vi "FPGA Target 2.vi"() -> ()   [LabVIEW 2019]
uses:
  <vilib>/Platform/TimedLoop/XDataNode/wakeup.ctl
  <vilib>/Platform/TimedLoop/XDataNode/XDNodeRunTimeDep.lvlib
  <vilib>/Platform/TimedLoop/XDataNode/nitl_modes.ctl
  <vilib>/Platform/TimedLoop/XDataNode/timing_clust.ctl
  <vilib>/Platform/TimedLoop/XDataNode/XDataNode.xnode
  SubModules/Engine Simulation Toolkit FPGA IP/IP Source/APU/APU.lvlib
  <vilib>/rvi/DataTransferAndStorage/Container/XNode/niFpgaContainer.xnode
  Templates/FPGA Wizard Templates.lvlib
  SubModules/Engine Simulation Toolkit FPGA IP/IP Source/Digital Pattern Generation/Digital Pattern Generation.lvlib
  SubModules/Engine Simulation Toolkit FPGA IP/IP Source/Directional Speed/Directional Speed.lvlib
  SubModules/FPGA Addon Speciality IO/Source/Speciality FPGA IO.lvlib
  SubModules/Engine Simulation Toolkit FPGA IP/IP Source/ECU Event/Timing/ECU Event Timing.lvlib
  SubModules/Engine Simulation Toolkit FPGA IP/IP Source/ECU Event/Timing/Measure Events (Non-40MHz).vi
  SubModules/Engine Simulation Toolkit FPGA IP/IP Source/ECU Event/Timing/Capture Settings.ctl
  <vilib>/rvi/interface/RandomDataEmulation/nirviRandomDataFpgaReadWriteTemplate.vi
  SubModules/Engine Simulation Toolkit FPGA IP/IP Source/APU/Shared Settings.ctl
  SubModules/Engine Simulation Toolkit FPGA IP/IP Source/Version Token.ctl
  SubModules/Engine Simulation Toolkit FPGA IP/IP Source/Engine Simulation Toolkit.lvlib
  SubModules/Engine Simulation Toolkit FPGA IP/IP Source/APU/Settings.ctl
  SubModules/Engine Simulation Toolkit FPGA IP/IP Source/APU/Input.ctl
  SubModules/Engine Simulation Toolkit FPGA IP/IP Source/APU/Output.ctl
  SubModules/Engine Simulation Toolkit FPGA IP/IP Source/Digital Pattern Generation/Load Input.ctl
  SubModules/Engine Simulation Toolkit FPGA IP/IP Source/Directional Speed/Load Input.ctl
  SubModules/FPGA Addon Speciality IO/Source/Types/PWM.Generate.Digital.Settings.ctl
  SubModules/FPGA Addon Speciality IO/Source/Types/PWM.Measure.Digital.Settings.ctl
  SubModules/FPGA Addon Speciality IO/Source/Types/PWM.Measure.Digital.Measurement.ctl
  SubModules/FPGA Addon Speciality IO/Source/Types/Static.Measure.Digital.Settings.ctl
  SubModules/FPGA Addon Speciality IO/Source/Types/Static.Measure.Digital.Measurement.ctl
  SubModules/FPGA Addon Speciality IO/Source/Types/Static.Generate.Digital.Settings.ctl
  SubModules/Engine Simulation Toolkit FPGA IP/IP Source/Digital Pattern Generation/Settings.ctl
  SubModules/Engine Simulation Toolkit FPGA IP/IP Source/Digital Pattern Generation/Input.ctl
  SubModules/FPGA Addon Speciality IO/Source/Types/WSS.Generate.Digital.Settings.ctl
  SubModules/Engine Simulation Toolkit FPGA IP/IP Source/Directional Speed/Settings.ctl
  SubModules/Engine Simulation Toolkit FPGA IP/IP Source/Directional Speed/Input.ctl
  SubModules/Engine Simulation Toolkit FPGA IP/IP Source/ECU Event/Timing/Measure Settings.ctl
  SubModules/Engine Simulation Toolkit FPGA IP/IP Source/ECU Event/Timing/Measure Output.ctl
  SubModules/Engine Simulation Toolkit FPGA IP/IP Source/ECU Event/Timing/Capture Output.ctl
panel:
  out "capture.Cyl Inj 2.Event 4":T1
  out "capture.Cyl Inj 2.Event 3":T1
  out "capture.Cyl Inj 2.Event 2":T1
  out "capture.Cyl Inj 2.Event 1":T1
  out "status.Cyl Inj 2":T2
  in  "settings.Cyl Inj 2":T3
  out "capture.Cyl Inj 1.Event 4":T1
  out "capture.Cyl Inj 1.Event 3":T1
  out "capture.Cyl Inj 1.Event 2":T1
  out "capture.Cyl Inj 1.Event 1":T1
  out "status.Cyl Inj 1":T2
  in  "settings.Cyl Inj 1":T3
  out "PWM IN 2.Measure":T4
  in  "PWM IN 2.Settings":T5={"ACTIVE EDGE"=TRUE, "TIMEOUT"=40000000}
  out "PWM IN 1.Measure":T4
  in  "PWM IN 1.Settings":T5={"ACTIVE EDGE"=TRUE, "TIMEOUT"=40000000}
  out "Mod2.Monitor":bool[](array[boolean])
  out "Mod1.Monitor":bool[](array[boolean])
  in  "input.Crank":T6
  in  "settings.Crank":T7
  in  "input.Crank_Temp":T8
  in  "settings.Crank_Temp":T9
  in  "Front Driver WS.Settings":T10={"ACTIVE EDGE"=TRUE, "ACTIVE TICKS"=0, "INACTIVE TICKS"=0, "DATA"=0, "SENSOR TYPE"=0}
  in  "input.Exhaust CAM 1":T8
  in  "settings.Exhaust CAM 1":T9
  in  "input.Intake CAM 1":T8
  in  "settings.Intake CAM 1":T9
  in  "PWM Out 2.Settings":T11={"ACTIVE EDGE"=TRUE, "ACTIVE TICKS"=0, "INACTIVE TICKS"=0}
  in  "PWM Out 1.Settings":T11={"ACTIVE EDGE"=TRUE, "ACTIVE TICKS"=0, "INACTIVE TICKS"=0}
  out "Mod9.Monitor":bool[](array[boolean])
  in  "Relay 103.Settings":T12={"ACTIVE EDGE"=TRUE, "OUTPUT"=FALSE}
  in  "Relay 102.Settings":T12={"ACTIVE EDGE"=TRUE, "OUTPUT"=FALSE}
  in  "Relay 101.Settings":T12={"ACTIVE EDGE"=TRUE, "OUTPUT"=FALSE}
  in  "Relay 100.Settings":T12={"ACTIVE EDGE"=TRUE, "OUTPUT"=FALSE}
  in  "Relay 99.Settings":T12={"ACTIVE EDGE"=TRUE, "OUTPUT"=FALSE}
  in  "Relay 98.Settings":T12={"ACTIVE EDGE"=TRUE, "OUTPUT"=FALSE}
  in  "Relay 97.Settings":T12={"ACTIVE EDGE"=TRUE, "OUTPUT"=FALSE}
  in  "Relay 96.Settings":T12={"ACTIVE EDGE"=TRUE, "OUTPUT"=FALSE}
  out "State 83.Measure":T13
  in  "State 83.Settings":T14={"ACTIVE EDGE"=TRUE}
  out "State 82.Measure":T13
  in  "State 82.Settings":T14={"ACTIVE EDGE"=TRUE}
  out "State 81.Measure":T13
  in  "State 81.Settings":T14={"ACTIVE EDGE"=TRUE}
  out "State 80.Measure":T13
  in  "State 80.Settings":T14={"ACTIVE EDGE"=TRUE}
  out "State 79.Measure":T13
  in  "State 79.Settings":T14={"ACTIVE EDGE"=TRUE}
  out "State 78.Measure":T13
  in  "State 78.Settings":T14={"ACTIVE EDGE"=TRUE}
  out "State 77.Measure":T13
  in  "State 77.Settings":T14={"ACTIVE EDGE"=TRUE}
  out "State 76.Measure":T13
  in  "State 76.Settings":T14={"ACTIVE EDGE"=TRUE}
  out "State 75.Measure":T13
  in  "State 75.Settings":T14={"ACTIVE EDGE"=TRUE}
  out "State 74.Measure":T13
  in  "State 74.Settings":T14={"ACTIVE EDGE"=TRUE}
  out "State 73.Measure":T13
  in  "State 73.Settings":T14={"ACTIVE EDGE"=TRUE}
  out "State 72.Measure":T13
  in  "State 72.Settings":T14={"ACTIVE EDGE"=TRUE}
  out "State 71.Measure":T13
  in  "State 71.Settings":T14={"ACTIVE EDGE"=TRUE}
  out "State 70.Measure":T13
  in  "State 70.Settings":T14={"ACTIVE EDGE"=TRUE}
  out "State 69.Measure":T13
  in  "State 69.Settings":T14={"ACTIVE EDGE"=TRUE}
  out "State 68.Measure":T13
  in  "State 68.Settings":T14={"ACTIVE EDGE"=TRUE}
  out "State 67.Measure":T13
  in  "State 67.Settings":T14={"ACTIVE EDGE"=TRUE}
  out "State 66.Measure":T13
  in  "State 66.Settings":T14={"ACTIVE EDGE"=TRUE}
  out "State 65.Measure":T13
  in  "State 65.Settings":T14={"ACTIVE EDGE"=TRUE}
  out "State 64.Measure":T13
  in  "State 64.Settings":T14={"ACTIVE EDGE"=TRUE}
  out "State 63.Measure":T13
  in  "State 63.Settings":T14={"ACTIVE EDGE"=TRUE}
  out "State 62.Measure":T13
  in  "State 62.Settings":T14={"ACTIVE EDGE"=TRUE}
  out "State 61.Measure":T13
  in  "State 61.Settings":T14={"ACTIVE EDGE"=TRUE}
  out "State 60.Measure":T13
  in  "State 60.Settings":T14={"ACTIVE EDGE"=TRUE}
  out "State 59.Measure":T13
  in  "State 59.Settings":T14={"ACTIVE EDGE"=TRUE}
  out "State 58.Measure":T13
  in  "State 58.Settings":T14={"ACTIVE EDGE"=TRUE}
  out "State 57.Measure":T13
  in  "State 57.Settings":T14={"ACTIVE EDGE"=TRUE}
  out "State 56.Measure":T13
  in  "State 56.Settings":T14={"ACTIVE EDGE"=TRUE}
  out "State 55.Measure":T13
  in  "State 55.Settings":T14={"ACTIVE EDGE"=TRUE}
  out "State 54.Measure":T13
  in  "State 54.Settings":T14={"ACTIVE EDGE"=TRUE}
  out "State 53.Measure":T13
  in  "State 53.Settings":T14={"ACTIVE EDGE"=TRUE}
  out "State 52.Measure":T13
  in  "State 52.Settings":T14={"ACTIVE EDGE"=TRUE}
  out "Mod8.Monitor":bool[](array[boolean])
  out "State 51.Measure":T13
  in  "State 51.Settings":T14={"ACTIVE EDGE"=TRUE}
  out "State 50.Measure":T13
  in  "State 50.Settings":T14={"ACTIVE EDGE"=TRUE}
  out "State 49.Measure":T13
  in  "State 49.Settings":T14={"ACTIVE EDGE"=TRUE}
  out "State 48.Measure":T13
  in  "State 48.Settings":T14={"ACTIVE EDGE"=TRUE}
  out "State 47.Measure":T13
  in  "State 47.Settings":T14={"ACTIVE EDGE"=TRUE}
  out "State 46.Measure":T13
  in  "State 46.Settings":T14={"ACTIVE EDGE"=TRUE}
  out "State 45.Measure":T13
  in  "State 45.Settings":T14={"ACTIVE EDGE"=TRUE}
  out "State 44.Measure":T13
  in  "State 44.Settings":T14={"ACTIVE EDGE"=TRUE}
  out "State 43.Measure":T13
  in  "State 43.Settings":T14={"ACTIVE EDGE"=TRUE}
  out "State 42.Measure":T13
  in  "State 42.Settings":T14={"ACTIVE EDGE"=TRUE}
  out "State 41.Measure":T13
  in  "State 41.Settings":T14={"ACTIVE EDGE"=TRUE}
  out "State 40.Measure":T13
  in  "State 40.Settings":T14={"ACTIVE EDGE"=TRUE}
  out "State 39.Measure":T13
  in  "State 39.Settings":T14={"ACTIVE EDGE"=TRUE}
  out "State 38.Measure":T13
  in  "State 38.Settings":T14={"ACTIVE EDGE"=TRUE}
  out "State 37.Measure":T13
  in  "State 37.Settings":T14={"ACTIVE EDGE"=TRUE}
  out "State 36.Measure":T13
  in  "State 36.Settings":T14={"ACTIVE EDGE"=TRUE}
  out "State 35.Measure":T13
  in  "State 35.Settings":T14={"ACTIVE EDGE"=TRUE}
  out "State 34.Measure":T13
  in  "State 34.Settings":T14={"ACTIVE EDGE"=TRUE}
  out "State 33.Measure":T13
  in  "State 33.Settings":T14={"ACTIVE EDGE"=TRUE}
  out "State 32.Measure":T13
  in  "State 32.Settings":T14={"ACTIVE EDGE"=TRUE}
  out "State 31.Measure":T13
  in  "State 31.Settings":T14={"ACTIVE EDGE"=TRUE}
  out "State 30.Measure":T13
  in  "State 30.Settings":T14={"ACTIVE EDGE"=TRUE}
  out "State 29.Measure":T13
  in  "State 29.Settings":T14={"ACTIVE EDGE"=TRUE}
  out "State 28.Measure":T13
  in  "State 28.Settings":T14={"ACTIVE EDGE"=TRUE}
  out "State 27":bool
  out "State 26":bool
  out "State 25":bool
  out "State 24":bool
  out "State 23":bool
  out "State 22":bool
  out "State 21":bool
  out "State 20":bool
  out "Mod7.Monitor":bool[](array[boolean])
  out "State 19":bool
  out "State 18":bool
  out "State 17":bool
  out "State 16":bool
  out "State 15":bool
  out "State 14":bool
  out "State 13":bool
  out "State 12":bool
  out "Mod6.Monitor":bool[](array[boolean])
  out "State 11":bool
  out "State 10":bool
  out "State 9":bool
  out "State 8":bool
  out "State 7":bool
  out "State 6":bool
  out "State 5":bool
  out "State 4":bool
  out "Mod5.Monitor":bool[](array[boolean])
  out "State 3":bool
  out "State 2":bool
  out "State 1":bool
  out "State 0":bool
  out "PWM IN 6.Measure":T4
  in  "PWM IN 6.Settings":T5={"ACTIVE EDGE"=TRUE, "TIMEOUT"=40000000}
  out "PWM IN 5.Measure":T4
  in  "PWM IN 5.Settings":T5={"ACTIVE EDGE"=TRUE, "TIMEOUT"=40000000}
  out "PWM IN 4.Measure":T4
  in  "PWM IN 4.Settings":T5={"ACTIVE EDGE"=TRUE, "TIMEOUT"=40000000}
  out "PWM IN 3.Measure":T4
  in  "PWM IN 3.Settings":T5={"ACTIVE EDGE"=TRUE, "TIMEOUT"=40000000}
  out "Mod4.Monitor":bool[](array[boolean])
  out "Mod3.Monitor":bool[](array[boolean])
  in  "Output 4":bool
  in  "Output 3":bool
  in  "Output 2":bool
  in  "Output 1":bool
  in  "Output 0":bool
  in  "PWM Out 27.Settings":T11={"ACTIVE EDGE"=TRUE, "ACTIVE TICKS"=0, "INACTIVE TICKS"=0}
  in  "PWM Out 26.Settings":T11={"ACTIVE EDGE"=TRUE, "ACTIVE TICKS"=0, "INACTIVE TICKS"=0}
  in  "PWM Out 25.Settings":T11={"ACTIVE EDGE"=TRUE, "ACTIVE TICKS"=0, "INACTIVE TICKS"=0}
  in  "PWM Out 24.Settings":T11={"ACTIVE EDGE"=TRUE, "ACTIVE TICKS"=0, "INACTIVE TICKS"=0}
  in  "PWM Out 23.Settings":T11={"ACTIVE EDGE"=TRUE, "ACTIVE TICKS"=0, "INACTIVE TICKS"=0}
  in  "PWM Out 22.Settings":T11={"ACTIVE EDGE"=TRUE, "ACTIVE TICKS"=0, "INACTIVE TICKS"=0}
  in  "PWM Out 21.Settings":T11={"ACTIVE EDGE"=TRUE, "ACTIVE TICKS"=0, "INACTIVE TICKS"=0}
  in  "PWM Out 20.Settings":T11={"ACTIVE EDGE"=TRUE, "ACTIVE TICKS"=0, "INACTIVE TICKS"=0}
  in  "PWM Out 19.Settings":T11={"ACTIVE EDGE"=TRUE, "ACTIVE TICKS"=0, "INACTIVE TICKS"=0}
  in  "PWM Out 18.Settings":T11={"ACTIVE EDGE"=TRUE, "ACTIVE TICKS"=0, "INACTIVE TICKS"=0}
  in  "PWM Out 17.Settings":T11={"ACTIVE EDGE"=TRUE, "ACTIVE TICKS"=0, "INACTIVE TICKS"=0}
  in  "PWM Out 16.Settings":T11={"ACTIVE EDGE"=TRUE, "ACTIVE TICKS"=0, "INACTIVE TICKS"=0}
  in  "PWM Out 15.Settings":T11={"ACTIVE EDGE"=TRUE, "ACTIVE TICKS"=0, "INACTIVE TICKS"=0}
  in  "PWM Out 14.Settings":T11={"ACTIVE EDGE"=TRUE, "ACTIVE TICKS"=0, "INACTIVE TICKS"=0}
  in  "PWM Out 13.Settings":T11={"ACTIVE EDGE"=TRUE, "ACTIVE TICKS"=0, "INACTIVE TICKS"=0}
  in  "PWM Out 12.Settings":T11={"ACTIVE EDGE"=TRUE, "ACTIVE TICKS"=0, "INACTIVE TICKS"=0}
  in  "PWM Out 11.Settings":T11={"ACTIVE EDGE"=TRUE, "ACTIVE TICKS"=0, "INACTIVE TICKS"=0}
  in  "PWM Out 10.Settings":T11={"ACTIVE EDGE"=TRUE, "ACTIVE TICKS"=0, "INACTIVE TICKS"=0}
  in  "PWM Out 9.Settings":T11={"ACTIVE EDGE"=TRUE, "ACTIVE TICKS"=0, "INACTIVE TICKS"=0}
  in  "PWM Out 8.Settings":T11={"ACTIVE EDGE"=TRUE, "ACTIVE TICKS"=0, "INACTIVE TICKS"=0}
  in  "PWM Out 7.Settings":T11={"ACTIVE EDGE"=TRUE, "ACTIVE TICKS"=0, "INACTIVE TICKS"=0}
  in  "PWM Out 6.Settings":T11={"ACTIVE EDGE"=TRUE, "ACTIVE TICKS"=0, "INACTIVE TICKS"=0}
  in  "PWM Out 5.Settings":T11={"ACTIVE EDGE"=TRUE, "ACTIVE TICKS"=0, "INACTIVE TICKS"=0}
  in  "PWM Out 4.Settings":T11={"ACTIVE EDGE"=TRUE, "ACTIVE TICKS"=0, "INACTIVE TICKS"=0}
  in  "PWM Out 3.Settings":T11={"ACTIVE EDGE"=TRUE, "ACTIVE TICKS"=0, "INACTIVE TICKS"=0}
  in  "PWM Out 2.Settings":T11={"ACTIVE EDGE"=TRUE, "ACTIVE TICKS"=0, "INACTIVE TICKS"=0}
  in  "PWM Out 1.Settings":T11={"ACTIVE EDGE"=TRUE, "ACTIVE TICKS"=0, "INACTIVE TICKS"=0}
  out "Mod14.Monitor":bool[](array[boolean])
  in  "Relay 95":bool
  in  "Relay 94":bool
  in  "Relay 93":bool
  in  "Relay 92":bool
  in  "Relay 91":bool
  in  "Relay 90":bool
  in  "Relay 89":bool
  in  "Relay 88":bool
  in  "Relay 87":bool
  in  "Relay 86":bool
  in  "Relay 85":bool
  in  "Relay 84":bool
  in  "Relay 83":bool
  in  "Relay 82":bool
  in  "Relay 81":bool
  in  "Relay 80":bool
  out "Mod13.Monitor":bool[](array[boolean])
  in  "Relay 79":bool
  in  "Relay 78":bool
  in  "Relay 77":bool
  in  "Relay 76":bool
  in  "Relay 75":bool
  in  "Relay 74":bool
  in  "Relay 73":bool
  in  "Relay 72":bool
  in  "Relay 71":bool
  in  "Relay 70":bool
  in  "Relay 69":bool
  in  "Relay 68":bool
  in  "Relay 67":bool
  in  "Relay 66":bool
  in  "Relay 65":bool
  in  "Relay 64":bool
  in  "Relay 63":bool
  in  "Relay 62":bool
  in  "Relay 61":bool
  in  "Relay 60":bool
  in  "Relay 59":bool
  in  "Relay 58":bool
  in  "Relay 57":bool
  in  "Relay 56":bool
  in  "Relay 55":bool
  in  "Relay 54":bool
  in  "Relay 53":bool
  in  "Relay 52":bool
  in  "Relay 51":bool
  in  "Relay 50":bool
  in  "Relay 49":bool
  in  "Relay 48":bool
  out "Mod12.Monitor":bool[](array[boolean])
  in  "Relay 47":bool
  in  "Relay 46":bool
  in  "Relay 45":bool
  in  "Relay 44":bool
  in  "Relay 43":bool
  in  "Relay 42":bool
  in  "Relay 41":bool
  in  "Relay 40":bool
  in  "Relay 39":bool
  in  "Relay 38":bool
  in  "Relay 37":bool
  in  "Relay 36":bool
  in  "Relay 35":bool
  in  "Relay 34":bool
  in  "Relay 33":bool
  in  "Relay 32":bool
  in  "Relay 31":bool
  in  "Relay 30":bool
  in  "Relay 29":bool
  in  "Relay 28":bool
  in  "Relay 27":bool
  in  "Relay 26":bool
  in  "Relay 25":bool
  in  "Relay 24":bool
  in  "Relay 23":bool
  in  "Relay 22":bool
  in  "Relay 21":bool
  in  "Relay 20":bool
  in  "Relay 19":bool
  in  "Relay 18":bool
  in  "Relay 17":bool
  in  "Relay 16":bool
  out "Mod11.Monitor":bool[](array[boolean])
  in  "Relay 15":bool
  in  "Relay 14":bool
  in  "Relay 13":bool
  in  "Relay 12":bool
  in  "Relay 11":bool
  in  "Relay 10":bool
  in  "Relay 9":bool
  in  "Relay 8":bool
  out "Mod10.Monitor":bool[](array[boolean])
  in  "Relay 7":bool
  in  "Relay 6":bool
  in  "Relay 5":bool
  in  "Relay 4":bool
  in  "Relay 3":bool
  in  "Relay 2":bool
  in  "Relay 1":bool
  in  "Relay 0":bool
  in  "load input.Crank":T15
  in  "load input.Crank_Temp":T16
  in  "load input.Exhaust CAM 1":T16
  in  "load input.Intake CAM 1":T16
  out "Actual Analog Input Loop Period (usec)":u32
  out "Actual Analog Output Loop Period (usec)":u32
  out "Actual Digital Loop Period (usec)":u32
  out "Actual DMA Loop Period (usec)":u32
  in  "Analog Input Loop Timer (uSec)":u32=10
  out "output.apu 1":T17 caption="output"
  in  "input.apu 1":T18={"desired speed"=0.0, "reset"=TRUE} caption="input"
  in  "settings.apu 1":T19 caption="settings"
  in  "est.version":T20
  in  "shared settings.apu 1":T21 {"start" format="%#.15g"}
  in  "go.apu 1":bool
  in  "Digital Loop Timer (uSec)":u32=10
  in  "Analog Output Loop Timer (uSec)":u32=10
  in  "DMA.Enable":bool
  in  "DMA.MinimumSamples":u32=100000 caption="DMA Loop Timer (uSec)"
  out "DMA.Timeout":bool
  in  "DMA.Timeout.Reset":bool
  in  "DMA Loop Timer (uSec)":u32=10
types:
  T1 = typedef "Engine Simulation Toolkit.lvlib/ECU Event Timing.lvlib/Capture Output.ctl" = cluster{"Start":u16, "End":u16, "Duration (tics)":fxp<+,18,18>, "Event present":bool}
  T2 = typedef "Engine Simulation Toolkit.lvlib/ECU Event Timing.lvlib/Measure Output.ctl" = cluster{"stuck active":bool, "window all active":bool, "window orphan start":bool, "window orphan end":bool}
  T3 = typedef "Engine Simulation Toolkit.lvlib/ECU Event Timing.lvlib/Measure Settings.ctl" = cluster{"max":u16, "min":u16, "active high":bool, "wrap":bool}
  T4 = typedef "Speciality FPGA IO.lvlib/PWM.Measure.Digital.Measurement.ctl" = cluster{"ACTIVE TICKS":u32, "INACTIVE TICKS":u32, "ACQ TICKS":u32}
  T5 = typedef "Speciality FPGA IO.lvlib/PWM.Measure.Digital.Settings.ctl" = cluster{"ACTIVE EDGE":bool, "TIMEOUT":u32}
  T6 = typedef "Engine Simulation Toolkit.lvlib/Directional Speed.lvlib/Input.ctl" = cluster{"td (tics)":u16, "tf (tics)":u16, "tr (tics)":u16}
  T7 = typedef "Engine Simulation Toolkit.lvlib/Directional Speed.lvlib/Settings.ctl" = cluster{"Upper Value":u16, "Lower Value":u16, "Upper Index":fxp<+,10,10>, "Lower Index":fxp<+,10,10>, "Enabled":bool}
  T8 = typedef "Engine Simulation Toolkit.lvlib/Digital Pattern Generation.lvlib/Input.ctl" = cluster{"Offset":i16}
  T9 = typedef "Engine Simulation Toolkit.lvlib/Digital Pattern Generation.lvlib/Settings.ctl" = cluster{"edge 1":u16, "edge 2":u16, "cycle angle":bool, "enabled":bool, "first falling":bool, "fault":bool, "fault wrap":bool, "fault value":bool, "fault count":fxp<+,4,4>, "use fault count":bool}
  T10 = typedef "Speciality FPGA IO.lvlib/WSS.Generate.Digital.Settings.ctl" = cluster{"ACTIVE EDGE":bool, "ACTIVE TICKS":u32, "INACTIVE TICKS":u32, "DATA":u8, "SENSOR TYPE":u8}
  T11 = typedef "Speciality FPGA IO.lvlib/PWM.Generate.Digital.Settings.ctl" = cluster{"ACTIVE EDGE":bool, "ACTIVE TICKS":u32, "INACTIVE TICKS":u32}
  T12 = typedef "Speciality FPGA IO.lvlib/Static.Generate.Digital.Settings.ctl" = cluster{"ACTIVE EDGE":bool, "OUTPUT":bool}
  T13 = typedef "Speciality FPGA IO.lvlib/Static.Measure.Digital.Measurement.ctl" = cluster{"STATE":bool}
  T14 = typedef "Speciality FPGA IO.lvlib/Static.Measure.Digital.Settings.ctl" = cluster{"ACTIVE EDGE":bool}
  T15 = typedef "Engine Simulation Toolkit.lvlib/Directional Speed.lvlib/Load Input.ctl" = cluster{"address":fxp<+,10,10>, "done":bool, "angle":u16}
  T16 = typedef "Engine Simulation Toolkit.lvlib/Digital Pattern Generation.lvlib/Load Input.ctl" = cluster{"address":fxp<+,11,11>, "done":bool, "angle":u16}
  T17 = typedef "Engine Simulation Toolkit.lvlib/APU.lvlib/Output.ctl" = cluster{"crank":u16, "cycle":u16, "actual speed":fxp<+/-,23,2>}
  T18 = typedef "Engine Simulation Toolkit.lvlib/APU.lvlib/Input.ctl" = cluster{"desired speed":fxp<+/-,23,2>, "reset":bool}
  T19 = typedef "Engine Simulation Toolkit.lvlib/APU.lvlib/Settings.ctl" = cluster{"acceleration":fxp<+,18,-20>, "enable accel":bool}
  T20 = typedef "Engine Simulation Toolkit.lvlib/Version Token.ctl" = cluster{"1.3.0":bool}
  T21 = typedef "Engine Simulation Toolkit.lvlib/APU.lvlib/Shared Settings.ctl" = cluster{"start":fxp<+,17,17>, "stuck limit":fxp<+,18,18>}
  T22 = typedef "XDNodeRunTimeDep.lvlib/timing_clust.ctl" = cluster{"Expected End [f-1]":u64, "Actual End [f-1]":u64, "Finished Late? [f-1]":bool, "Expected End [i-1]":u64, "Actual End [i-1]":u64, "Finished Late? [i-1]":bool, "Expected Start [i]":u64, "Actual Start [i]":u64, "Expected Start [f]":u64, "Actual Start [f]":u64, "Source Name":string, "Structure Name":string, "Period":i64, "Deadline":i64, "Offset":i64, "Start":i64, "Priority":i32, "Timeout":i32, "Mode":T23, "Wakeup Reason":T24, "Error":errorcluster, "Source Type":string, "Secondary Source Type":string, "Global End Time":u64, "Global Start Time":u64, "Frame Duration":u64, "Iteration Duration":u64, "Assigned CPU":i32, "I/O Scan Engine Mode":u32}
  T23 = typedef "XDNodeRunTimeDep.lvlib/nitl_modes.ctl" = enum32{"No Change", "Process missed periods, maintain original phase", "Discard missed periods, maintain original phase", "Process missed periods, ignore original phase", "Discard missed periods, ignore original phase"}
  T24 = typedef "XDNodeRunTimeDep.lvlib/wakeup.ctl" = enum32{"Normal", "Aborted", "Asynchronous wakeup", "Timing source error", "Timed loop error", "Timeout"}
  T25 = typedef "Engine Simulation Toolkit.lvlib/ECU Event Timing.lvlib/Capture Settings.ctl" = u8
  T26 = cluster{"DI 0":refnum<k21>, "DI 1":refnum<k21>, "DI 2":refnum<k21>, "DI 3":refnum<k21>}
  T27 = cluster{"DO 0":refnum<k21>, "DO 1":refnum<k21>, "DO 2":refnum<k21>, "DO 3":refnum<k21>, "DO 4":refnum<k21>, "DO 5":refnum<k21>, "DO 6":refnum<k21>, "DO 7":refnum<k21>}
  T28 = cluster{"DI 0":refnum<k21>, "DI 1":refnum<k21>, "DI 2":refnum<k21>, "DI 3":refnum<k21>, "DI 4":refnum<k21>, "DI 5":refnum<k21>, "DI 6":refnum<k21>, "DI 7":refnum<k21>, "DI 8":refnum<k21>, "DI 9":refnum<k21>, "DI 10":refnum<k21>, "DI 11":refnum<k21>, "DI 12":refnum<k21>, "DI 13":refnum<k21>, "DI 14":refnum<k21>, "DI 15":refnum<k21>, "DI 16":refnum<k21>, "DI 17":refnum<k21>, "DI 18":refnum<k21>, "DI 19":refnum<k21>, "DI 20":refnum<k21>, "DI 21":refnum<k21>, "DI 22":refnum<k21>, "DI 23":refnum<k21>, "DI 24":refnum<k21>, "DI 25":refnum<k21>, "DI 26":refnum<k21>, "DI 27":refnum<k21>, "DI 28":refnum<k21>, "DI 29":refnum<k21>, "DI 30":refnum<k21>, "DI 31":refnum<k21>}
  T29 = cluster{"DI 0":refnum<k21>, "DI 1":refnum<k21>, "DI 2":refnum<k21>, "DI 3":refnum<k21>, "DI 4":refnum<k21>, "DI 5":refnum<k21>, "DI 6":refnum<k21>, "DI 7":refnum<k21>}
  T30 = cluster{"DO 0":refnum<k21>, "DO 1":refnum<k21>, "DO 2":refnum<k21>, "DO 3":refnum<k21>, "DO 4":refnum<k21>, "DO 5":refnum<k21>, "DO 6":refnum<k21>, "DO 7":refnum<k21>, "DO 8":refnum<k21>, "DO 9":refnum<k21>, "DO 10":refnum<k21>, "DO 11":refnum<k21>, "DO 12":refnum<k21>, "DO 13":refnum<k21>, "DO 14":refnum<k21>, "DO 15":refnum<k21>, "DO 16":refnum<k21>, "DO 17":refnum<k21>, "DO 18":refnum<k21>, "DO 19":refnum<k21>, "DO 20":refnum<k21>, "DO 21":refnum<k21>, "DO 22":refnum<k21>, "DO 23":refnum<k21>, "DO 24":refnum<k21>, "DO 25":refnum<k21>, "DO 26":refnum<k21>, "DO 27":refnum<k21>, "DO 28":refnum<k21>, "DO 29":refnum<k21>, "DO 30":refnum<k21>, "DO 31":refnum<k21>}
  T31 = cluster{"DO 0":refnum<k21>, "DO 1":refnum<k21>, "DO 2":refnum<k21>, "DO 3":refnum<k21>, "DO 4":refnum<k21>, "DO 5":refnum<k21>, "DO 6":refnum<k21>, "DO 7":refnum<k21>, "DO 8":refnum<k21>, "DO 9":refnum<k21>, "DO 10":refnum<k21>, "DO 11":refnum<k21>, "DO 12":refnum<k21>, "DO 13":refnum<k21>, "DO 14":refnum<k21>, "DO 15":refnum<k21>}
  T32 = typedef "Engine Simulation Toolkit.lvlib/Digital Pattern Generation.lvlib/Load Data.ctl" = cluster{"max address":fxp<+,11,11>, "memory":refnum<k21>}
  T33 = typedef "Engine Simulation Toolkit.lvlib/Directional Speed.lvlib/Load Data.ctl" = cluster{"max address":fxp<+,10,10>, "Memory":refnum<k21>}
  T34 = typedef "Engine Simulation Toolkit.lvlib/APU.lvlib/Register Bus.ctl" = cluster{"Speed":refnum<k21>, "Crank Angle":refnum<k21>, "Cycle Angle":refnum<k21>, "Crank Count":refnum<k21>, "Cycle Count":refnum<k21>, "1.25 MHz Counter":refnum<k21>, "Crank Rollover":refnum<k21>, "Cycle Rollover":refnum<k21>, "shared settings":T21}
  T35 = typedef "Engine Simulation Toolkit.lvlib/ECU Event Timing.lvlib/Measured Data.ctl" = cluster{"start":u16, "end":u16, "duration (tics)":fxp<+,18,18>, "window end":bool, "window begin":bool, "pulse end":bool, "pulse #":u8}
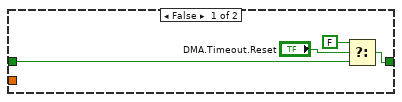
[diagram p2: hidden frame]
diagram:
  n1 = flat-sequence "Main Sequence Structure" {
    tunnel: [w18] -> w5
    tunnel: [w9] -> w4
    tunnel: [w8] -> w3
    tunnel: [w7] -> w2
    tunnel: [w6] -> w1
    tunnel: w5 -> [w70]
    tunnel: w4 -> [w69]
    tunnel: w3 -> [w68]
    tunnel: w2 -> [w67]
    tunnel: w1 -> [w66]
    frame #0 {
      n2 = node-c288() -> (w17:T22)  [unwired: 1 in]
      n3 = node-c288() -> (w15:T22)  [unwired: 1 in]
      n4 = node-c288() -> (w13:T22)  [unwired: 1 in]
      n5 = node-c288() -> (w11:T22)  [unwired: 1 in]
      n6 = node-c288() -> (w20:T22)  [unwired: 1 in]
      n7 = timed-loop "Intake CAM 1" {
        timing: w17 -> [_]
        timing-out: [_] -> w16
        tunnel: [w50] -> w9
        stop <- w53 stop-if-true
        n8 = call "Memory.Digital.Selection.vi"("memory"=refnum<k21> "Intake CAM 1") -> ("memory"=w51:refnum<k21>)  [unwired: 10 in]
        n9 = call "Load Digital Pattern Generation.vi"("memory"=w51, "load input.<user name>"="load input.Intake CAM 1") -> ("done"=w53:bool, "load data"=w50:T32)  [unwired: 8 in]
      }
      n10 = timed-loop "Exhaust CAM 1" {
        timing: w15 -> [_]
        timing-out: [_] -> w14
        tunnel: [w41] -> w8
        stop <- w44 stop-if-true
        n11 = call "Memory.Digital.Selection.vi"("memory"=refnum<k21> "Exhaust CAM 1") -> ("memory"=w42:refnum<k21>)  [unwired: 10 in]
        n12 = call "Load Digital Pattern Generation.vi"("memory"=w42, "load input.<user name>"="load input.Exhaust CAM 1") -> ("done"=w44:bool, "load data"=w41:T32)  [unwired: 8 in]
      }
      n13 = timed-loop "Crank_Temp" {
        timing: w13 -> [_]
        timing-out: [_] -> w12
        tunnel: [w32] -> w7
        stop <- w35 stop-if-true
        n14 = call "Memory.Digital.Selection.vi"("memory"=refnum<k21> "Crank_Temp") -> ("memory"=w33:refnum<k21>)  [unwired: 10 in]
        n15 = call "Load Digital Pattern Generation.vi"("memory"=w33, "load input.<user name>"="load input.Crank_Temp") -> ("done"=w35:bool, "load data"=w32:T32)  [unwired: 8 in]
      }
      n16 = timed-loop "Crank" {
        timing: w11 -> [_]
        timing-out: [_] -> w10
        tunnel: [w23] -> w6
        stop <- w26 stop-if-true
        n17 = call "Memory.Digital.Selection.vi"("memory"=refnum<k21> "Crank") -> ("memory"=w24:refnum<k21>)  [unwired: 10 in]
        n18 = call "Load Directional Speed Sensor.vi"("Memory In"=w24, "load input.<user name>"="load input.Crank") -> ("done"=w26:bool, "load data"=w23:T33)  [unwired: 8 in]
      }
      n19 = timed-loop "EST APU Init" {
        timing: w20 -> [_]
        timing-out: [_] -> w19
        tunnel: [w59] -> w18
        stop <- "go.apu 1" stop-if-true
        n20 = call "Create APU Register Bus.vi"("shared settings.<user name>"="shared settings.apu 1") -> ("register bus"=w59:T34)  [unwired: 10 in]
      }
      n21 = call <vilib>:"niFPGA Interrupt.vi"("Wait Until Cleared (F)"=TRUE, "IRQ Number (0)"=u8 30) -> ()  [unwired: 1 in]
      n22 = node-c288(w19) -> ()
      n23 = node-c288(w16) -> ()
      n24 = node-c288(w14) -> ()
      n25 = node-c288(w12) -> ()
      n26 = node-c288(w10) -> ()
    }
    frame #1 {
      # "FPGA Addon Code"
      n27 = node-c288 ("Input Node")() -> (w72:T22)  [unwired: 1 in]
      n28 = while "DMA Loop" {
        stop <- FALSE stop-if-true
        n29 = flat-sequence "Timing Control" {
          tunnel: [w153] -> w151
          tunnel: w151 -> [w197]
          frame #0 {
            n30 = call "Loop.Timer.vi"("Loop Timer (uSec)"="DMA Loop Timer (uSec)") -> ("Actual Loop Period (usec)"=w153:u32)  [unwired: 10 in]
          }
          frame #1 {
            n31 = local read "Mod10.Monitor"() -> (w196:bool[])
            n32 = local read "Mod11.Monitor"() -> (w194:bool[])
            n33 = local read "Mod12.Monitor"() -> (w192:bool[])
            n34 = local read "Mod13.Monitor"() -> (w190:bool[])
            n35 = local read "Mod14.Monitor"() -> (w188:bool[])
            n36 = local read "Mod3.Monitor"() -> (w186:bool[])
            n37 = local read "Mod4.Monitor"() -> (w184:bool[])
            n38 = local read "Mod5.Monitor"() -> (w182:bool[])
            n39 = local read "Mod6.Monitor"() -> (w180:bool[])
            n40 = local read "Mod7.Monitor"() -> (w178:bool[])
            n41 = local read "Mod8.Monitor"() -> (w176:bool[])
            n42 = local read "Mod9.Monitor"() -> (w174:bool[])
            n43 = local read "Mod1.Monitor"() -> (w172:bool[])
            n44 = local read "Mod2.Monitor"() -> (w170:bool[])
            n45 = Boolean To (0,1)(Boolean=w196) -> (0, 1=w195:i16[])
            n46 = Boolean To (0,1)(Boolean=w194) -> (0, 1=w193:i16[])
            n47 = Boolean To (0,1)(Boolean=w192) -> (0, 1=w191:i16[])
            n48 = Boolean To (0,1)(Boolean=w190) -> (0, 1=w189:i16[])
            n49 = Boolean To (0,1)(Boolean=w188) -> (0, 1=w187:i16[])
            n50 = Boolean To (0,1)(Boolean=w186) -> (0, 1=w185:i16[])
            n51 = Boolean To (0,1)(Boolean=w184) -> (0, 1=w183:i16[])
            n52 = Boolean To (0,1)(Boolean=w182) -> (0, 1=w181:i16[])
            n53 = Boolean To (0,1)(Boolean=w180) -> (0, 1=w179:i16[])
            n54 = Boolean To (0,1)(Boolean=w178) -> (0, 1=w177:i16[])
            n55 = Boolean To (0,1)(Boolean=w176) -> (0, 1=w175:i16[])
            n56 = Boolean To (0,1)(Boolean=w174) -> (0, 1=w173:i16[])
            n57 = Boolean To (0,1)(Boolean=w172) -> (0, 1=w171:i16[])
            n58 = Boolean To (0,1)(Boolean=w170) -> (0, 1=w169:i16[])
            n59 = To Single Precision Float(number=w195) -> (single precision float=w168:sgl[])
            n60 = To Single Precision Float(number=w193) -> (single precision float=w167:sgl[])
            n61 = To Single Precision Float(number=w191) -> (single precision float=w166:sgl[])
            n62 = To Single Precision Float(number=w189) -> (single precision float=w165:sgl[])
            n63 = To Single Precision Float(number=w187) -> (single precision float=w164:sgl[])
            n64 = To Single Precision Float(number=w185) -> (single precision float=w163:sgl[])
            n65 = To Single Precision Float(number=w183) -> (single precision float=w162:sgl[])
            n66 = To Single Precision Float(number=w181) -> (single precision float=w161:sgl[])
            n67 = To Single Precision Float(number=w179) -> (single precision float=w160:sgl[])
            n68 = To Single Precision Float(number=w177) -> (single precision float=w159:sgl[])
            n69 = To Single Precision Float(number=w175) -> (single precision float=w158:sgl[])
            n70 = To Single Precision Float(number=w173) -> (single precision float=w157:sgl[])
            n71 = To Single Precision Float(number=w171) -> (single precision float=w156:sgl[])
            n72 = To Single Precision Float(number=w169) -> (single precision float=w155:sgl[])
            n73 = Build Array (concatenate) "Build Array"(w168, w167, w166, w165, w164, w163, w162, w161, w160, w159, w158, w157, w156, w155) -> (w203:sgl[])
            n74 = call "DMA.Command.Handler.vi"("DMA.Enable"="DMA.Enable", "DMA.MinimumSamples"="DMA.MinimumSamples") -> ("Transfer"=w199:bool)  [unwired: 9 in]
            n75 = feedback #1() -> (w202:sgl[])  [unwired: 1 in]
            n76 = feedback-in #1(w203) -> ()
            n77 = feedback #2(FALSE ("t")) -> (w198:bool)
            n78 = case shown="True" w199 {
              tunnel: w202 -> [_ w212]
              tunnel: w198 -> [w207 w211]
              tunnel: [w206 w210] -> w201
              frame False {
                n79 = Select(t=FALSE, s="DMA.Timeout.Reset", f=w207) -> (s? t:f=w206:bool)
              }
              frame True {
                n80 = for {
                  shift-right: [w215] -> w210
                  shift-left: w211 -> [w214]
                  tunnel: w212 -> [w213] mode=indexing
                  n81 = xnode ("FIFO Method Node")("Element"=w213, "Timeout"=0) -> ("Timed Out?"=w216:bool)  [unwired: 1 in, 1 out]
                  n82 = Or(x=w214, y=w216) -> (x .or. y?=w215:bool)
                }
              }
            }
            "DMA.Timeout" <- w201
            n83 = feedback-in #2(w201) -> ()
            "Actual DMA Loop Period (usec)" <- w197
          }
        }
      }
      n84 = while "Digital Low Speed Loop" {
        tunnel: w70 -> [w236]
        stop <- FALSE stop-if-true
        n85 = flat-sequence "Timing Control" {
          tunnel: w236 -> [w643]
          tunnel: [w643] -> w235
          tunnel: [w641] -> w234
          tunnel: w235 -> [_]
          tunnel: w234 -> [w644]
          frame #0 {
            n86 = Build Array("Relay 48", "Relay 49", "Relay 50", "Relay 51", "Relay 52", "Relay 53", "Relay 54", "Relay 55", "Relay 56", "Relay 57", "Relay 58", "Relay 59", "Relay 60", "Relay 61", "Relay 62", "Relay 63", "Relay 64", "Relay 65", "Relay 66", "Relay 67", "Relay 68", "Relay 69", "Relay 70", "Relay 71", "Relay 72", "Relay 73", "Relay 74", "Relay 75", "Relay 76", "Relay 77", "Relay 78", "Relay 79") -> (w553:bool[])
            "Mod13.Monitor" <- w553
            n87 = Build Array("Relay 16", "Relay 17", "Relay 18", "Relay 19", "Relay 20", "Relay 21", "Relay 22", "Relay 23", "Relay 24", "Relay 25", "Relay 26", "Relay 27", "Relay 28", "Relay 29", "Relay 30", "Relay 31", "Relay 32", "Relay 33", "Relay 34", "Relay 35", "Relay 36", "Relay 37", "Relay 38", "Relay 39", "Relay 40", "Relay 41", "Relay 42", "Relay 43", "Relay 44", "Relay 45", "Relay 46", "Relay 47") -> (w587:bool[])
            "Mod12.Monitor" <- w587
            n88 = Build Array("Relay 80", "Relay 81", "Relay 82", "Relay 83", "Relay 84", "Relay 85", "Relay 86", "Relay 87", "Relay 88", "Relay 89", "Relay 90", "Relay 91", "Relay 92", "Relay 93", "Relay 94", "Relay 95") -> (w535:bool[])
            "Mod14.Monitor" <- w535
            n89 = Build Array("Relay 0", "Relay 1", "Relay 2", "Relay 3", "Relay 4", "Relay 5", "Relay 6", "Relay 7") -> (w631:bool[])
            "Mod10.Monitor" <- w631
            n90 = Build Array("Relay 8", "Relay 9", "Relay 10", "Relay 11", "Relay 12", "Relay 13", "Relay 14", "Relay 15") -> (w621:bool[])
            "Mod11.Monitor" <- w621
            n91 = call "Digital_Input_8Channels.vi"("IO"=T29 {"DI 0"="Mod6/DI0", "DI 1"="Mod6/DI1", "DI 2"="Mod6/DI2", "DI 3"="Mod6/DI3", "DI 4"="Mod6/DI4", "DI 5"="Mod6/DI5", "DI 6"="Mod6/DI6", "DI 7"="Mod6/DI7"}) -> ("States"=w444:bool[])
            "Mod6.Monitor" <- w444
            n92 = call "Digital_Input_8Channels.vi"("IO"=T29 {"DI 0"="Mod5/DI0", "DI 1"="Mod5/DI1", "DI 2"="Mod5/DI2", "DI 3"="Mod5/DI3", "DI 4"="Mod5/DI4", "DI 5"="Mod5/DI5", "DI 6"="Mod5/DI6", "DI 7"="Mod5/DI7"}) -> ("States"=w454:bool[])
            "Mod5.Monitor" <- w454
            n93 = call "Digital_Input_8Channels.vi"("IO"=T29 {"DI 0"="Mod4/DI0", "DI 1"="Mod4/DI1", "DI 2"="Mod4/DI2", "DI 3"="Mod4/DI3", "DI 4"="Mod4/DI4", "DI 5"="Mod4/DI5", "DI 6"="Mod4/DI6", "DI 7"="Mod4/DI7"}) -> ("States"=w472:bool[])
            "Mod4.Monitor" <- w472
            n94 = call "Digital_Output_8Channels.vi"("States"=w631, "IO"=T27 {"DO 0"="Mod10/DO0", "DO 1"="Mod10/DO1", "DO 2"="Mod10/DO2", "DO 3"="Mod10/DO3", "DO 4"="Mod10/DO4", "DO 5"="Mod10/DO5", "DO 6"="Mod10/DO6", "DO 7"="Mod10/DO7"}) -> ()  [unwired: 1 in]
            n95 = Index Array(array=w444) -> (element #1=→"State 12":bool, element #2=→"State 13":bool, element #3=→"State 14":bool, element #4=→"State 15":bool, element #5=→"State 16":bool, element #6=→"State 17":bool, element #7=→"State 18":bool, element #8=→"State 19":bool)  [unwired: 8 in]
            n96 = call "Digital_Output_8Channels.vi"("States"=w621, "IO"=T27 {"DO 0"="Mod11/DO0", "DO 1"="Mod11/DO1", "DO 2"="Mod11/DO2", "DO 3"="Mod11/DO3", "DO 4"="Mod11/DO4", "DO 5"="Mod11/DO5", "DO 6"="Mod11/DO6", "DO 7"="Mod11/DO7"}) -> ()  [unwired: 1 in]
            n97 = Index Array(array=w454) -> (element #1=→"State 4":bool, element #2=→"State 5":bool, element #3=→"State 6":bool, element #4=→"State 7":bool, element #5=→"State 8":bool, element #6=→"State 9":bool, element #7=→"State 10":bool, element #8=→"State 11":bool)  [unwired: 8 in]
            n98 = call "Static.Generate.Digital.vi"("Settings"="Relay 96.Settings") -> ("Output"=w247:bool)  [unwired: 10 in]
            n99 = call "Static.Generate.Digital.vi"("Settings"="Relay 97.Settings") -> ("Output"=w246:bool)  [unwired: 10 in]
            n100 = call "Static.Generate.Digital.vi"("Settings"="Relay 98.Settings") -> ("Output"=w245:bool)  [unwired: 10 in]
            n101 = call "Static.Generate.Digital.vi"("Settings"="Relay 99.Settings") -> ("Output"=w244:bool)  [unwired: 10 in]
            n102 = call "Static.Generate.Digital.vi"("Settings"="Relay 100.Settings") -> ("Output"=w243:bool)  [unwired: 10 in]
            n103 = call "Static.Generate.Digital.vi"("Settings"="Relay 101.Settings") -> ("Output"=w242:bool)  [unwired: 10 in]
            n104 = call "Static.Generate.Digital.vi"("Settings"="Relay 102.Settings") -> ("Output"=w241:bool)  [unwired: 10 in]
            n105 = call "Static.Generate.Digital.vi"("Settings"="Relay 103.Settings") -> ("Output"=w240:bool)  [unwired: 10 in]
            n106 = call "Digital_Output_32Channels.vi"("States"=w553, "IO"=T30 {"DO 0"="Mod13/DO0", "DO 1"="Mod13/DO1", "DO 2"="Mod13/DO2", "DO 3"="Mod13/DO3", "DO 4"="Mod13/DO4", "DO 5"="Mod13/DO5", "DO 6"="Mod13/DO6", "DO 7"="Mod13/DO7", "DO 8"="Mod13/DO8", "DO 9"="Mod13/DO9", "DO 10"="Mod13/DO10", "DO 11"="Mod13/DO11", "DO 12"="Mod13/DO12", "DO 13"="Mod13/DO13", "DO 14"="Mod13/DO14", "DO 15"="Mod13/DO15", "DO 16"="Mod13/DO16", "DO 17"="Mod13/DO17", "DO 18"="Mod13/DO18", "DO 19"="Mod13/DO19", "DO 20"="Mod13/DO20", "DO 21"="Mod13/DO21", "DO 22"="Mod13/DO22", "DO 23"="Mod13/DO23", "DO 24"="Mod13/DO24", "DO 25"="Mod13/DO25", "DO 26"="Mod13/DO26", "DO 27"="Mod13/DO27", "DO 28"="Mod13/DO28", "DO 29"="Mod13/DO29", "DO 30"="Mod13/DO30", "DO 31"="Mod13/DO31"}) -> ()  [unwired: 1 in]
            n107 = call "Digital_Output_16Channels.vi"("States"=w535, "IO"=T31 {"DO 0"="Mod14/DO0", "DO 1"="Mod14/DO1", "DO 2"="Mod14/DO2", "DO 3"="Mod14/DO3", "DO 4"="Mod14/DO4", "DO 5"="Mod14/DO5", "DO 6"="Mod14/DO6", "DO 7"="Mod14/DO7", "DO 8"="Mod14/DO8", "DO 9"="Mod14/DO9", "DO 10"="Mod14/DO10", "DO 11"="Mod14/DO11", "DO 12"="Mod14/DO12", "DO 13"="Mod14/DO13", "DO 14"="Mod14/DO14", "DO 15"="Mod14/DO15"}) -> ()  [unwired: 1 in]
            n108 = call "Digital_Output_32Channels.vi"("States"=w587, "IO"=T30 {"DO 0"="Mod12/DO0", "DO 1"="Mod12/DO1", "DO 2"="Mod12/DO2", "DO 3"="Mod12/DO3", "DO 4"="Mod12/DO4", "DO 5"="Mod12/DO5", "DO 6"="Mod12/DO6", "DO 7"="Mod12/DO7", "DO 8"="Mod12/DO8", "DO 9"="Mod12/DO9", "DO 10"="Mod12/DO10", "DO 11"="Mod12/DO11", "DO 12"="Mod12/DO12", "DO 13"="Mod12/DO13", "DO 14"="Mod12/DO14", "DO 15"="Mod12/DO15", "DO 16"="Mod12/DO16", "DO 17"="Mod12/DO17", "DO 18"="Mod12/DO18", "DO 19"="Mod12/DO19", "DO 20"="Mod12/DO20", "DO 21"="Mod12/DO21", "DO 22"="Mod12/DO22", "DO 23"="Mod12/DO23", "DO 24"="Mod12/DO24", "DO 25"="Mod12/DO25", "DO 26"="Mod12/DO26", "DO 27"="Mod12/DO27", "DO 28"="Mod12/DO28", "DO 29"="Mod12/DO29", "DO 30"="Mod12/DO30", "DO 31"="Mod12/DO31"}) -> ()  [unwired: 1 in]
            n109 = call "Digital_Input_32Channels.vi"("IO"=T28 {"DI 0"="Mod8/DI0", "DI 1"="Mod8/DI1", "DI 2"="Mod8/DI2", "DI 3"="Mod8/DI3", "DI 4"="Mod8/DI4", "DI 5"="Mod8/DI5", "DI 6"="Mod8/DI6", "DI 7"="Mod8/DI7", "DI 8"="Mod8/DI8", "DI 9"="Mod8/DI9", "DI 10"="Mod8/DI10", "DI 11"="Mod8/DI11", "DI 12"="Mod8/DI12", "DI 13"="Mod8/DI13", "DI 14"="Mod8/DI14", "DI 15"="Mod8/DI15", "DI 16"="Mod8/DI16", "DI 17"="Mod8/DI17", "DI 18"="Mod8/DI18", "DI 19"="Mod8/DI19", "DI 20"="Mod8/DI20", "DI 21"="Mod8/DI21", "DI 22"="Mod8/DI22", "DI 23"="Mod8/DI23", "DI 24"="Mod8/DI24", "DI 25"="Mod8/DI25", "DI 26"="Mod8/DI26", "DI 27"="Mod8/DI27", "DI 28"="Mod8/DI28", "DI 29"="Mod8/DI29", "DI 30"="Mod8/DI30", "DI 31"="Mod8/DI31"}) -> ("States"=w352:bool[])
            "Mod8.Monitor" <- w352
            n110 = Index Array(array=w472) -> (element #1=w470:bool, element #2=w467:bool, element #3=w464:bool, element #4=w461:bool, element #5=→"State 0":bool, element #6=→"State 1":bool, element #7=→"State 2":bool, element #8=→"State 3":bool)  [unwired: 8 in]
            n111 = call "Digital_Input_32Channels.vi"("IO"=T28 {"DI 0"="Mod7/DI0", "DI 1"="Mod7/DI1", "DI 2"="Mod7/DI2", "DI 3"="Mod7/DI3", "DI 4"="Mod7/DI4", "DI 5"="Mod7/DI5", "DI 6"="Mod7/DI6", "DI 7"="Mod7/DI7", "DI 8"="Mod7/DI8", "DI 9"="Mod7/DI9", "DI 10"="Mod7/DI10", "DI 11"="Mod7/DI11", "DI 12"="Mod7/DI12", "DI 13"="Mod7/DI13", "DI 14"="Mod7/DI14", "DI 15"="Mod7/DI15", "DI 16"="Mod7/DI16", "DI 17"="Mod7/DI17", "DI 18"="Mod7/DI18", "DI 19"="Mod7/DI19", "DI 20"="Mod7/DI20", "DI 21"="Mod7/DI21", "DI 22"="Mod7/DI22", "DI 23"="Mod7/DI23", "DI 24"="Mod7/DI24", "DI 25"="Mod7/DI25", "DI 26"="Mod7/DI26", "DI 27"="Mod7/DI27", "DI 28"="Mod7/DI28", "DI 29"="Mod7/DI29", "DI 30"="Mod7/DI30", "DI 31"="Mod7/DI31"}) -> ("States"=w434:bool[])
            "Mod7.Monitor" <- w434
            n112 = call "PWM.Generate.Digital.vi"("Settings"="PWM Out 1.Settings") -> ("Output"=w507:bool)  [unwired: 10 in]
            n113 = call "PWM.Generate.Digital.vi"("Settings"="PWM Out 2.Settings") -> ("Output"=w506:bool)  [unwired: 10 in]
            n114 = call "PWM.Generate.Digital.vi"("Settings"="PWM Out 3.Settings") -> ("Output"=w505:bool)  [unwired: 10 in]
            n115 = call "PWM.Generate.Digital.vi"("Settings"="PWM Out 4.Settings") -> ("Output"=w504:bool)  [unwired: 10 in]
            n116 = call "PWM.Generate.Digital.vi"("Settings"="PWM Out 5.Settings") -> ("Output"=w503:bool)  [unwired: 10 in]
            n117 = call "PWM.Generate.Digital.vi"("Settings"="PWM Out 6.Settings") -> ("Output"=w502:bool)  [unwired: 10 in]
            n118 = call "PWM.Generate.Digital.vi"("Settings"="PWM Out 7.Settings") -> ("Output"=w501:bool)  [unwired: 10 in]
            n119 = call "PWM.Generate.Digital.vi"("Settings"="PWM Out 8.Settings") -> ("Output"=w500:bool)  [unwired: 10 in]
            n120 = call "PWM.Generate.Digital.vi"("Settings"="PWM Out 9.Settings") -> ("Output"=w499:bool)  [unwired: 10 in]
            n121 = call "PWM.Generate.Digital.vi"("Settings"="PWM Out 10.Settings") -> ("Output"=w498:bool)  [unwired: 10 in]
            n122 = call "PWM.Generate.Digital.vi"("Settings"="PWM Out 11.Settings") -> ("Output"=w497:bool)  [unwired: 10 in]
            n123 = call "PWM.Generate.Digital.vi"("Settings"="PWM Out 12.Settings") -> ("Output"=w496:bool)  [unwired: 10 in]
            n124 = call "PWM.Generate.Digital.vi"("Settings"="PWM Out 13.Settings") -> ("Output"=w495:bool)  [unwired: 10 in]
            n125 = call "PWM.Generate.Digital.vi"("Settings"="PWM Out 14.Settings") -> ("Output"=w494:bool)  [unwired: 10 in]
            n126 = call "PWM.Generate.Digital.vi"("Settings"="PWM Out 15.Settings") -> ("Output"=w493:bool)  [unwired: 10 in]
            n127 = call "PWM.Generate.Digital.vi"("Settings"="PWM Out 16.Settings") -> ("Output"=w492:bool)  [unwired: 10 in]
            n128 = call "PWM.Generate.Digital.vi"("Settings"="PWM Out 17.Settings") -> ("Output"=w491:bool)  [unwired: 10 in]
            n129 = call "PWM.Generate.Digital.vi"("Settings"="PWM Out 18.Settings") -> ("Output"=w490:bool)  [unwired: 10 in]
            n130 = call "PWM.Generate.Digital.vi"("Settings"="PWM Out 19.Settings") -> ("Output"=w489:bool)  [unwired: 10 in]
            n131 = call "PWM.Generate.Digital.vi"("Settings"="PWM Out 20.Settings") -> ("Output"=w488:bool)  [unwired: 10 in]
            n132 = call "PWM.Generate.Digital.vi"("Settings"="PWM Out 21.Settings") -> ("Output"=w487:bool)  [unwired: 10 in]
            n133 = call "PWM.Generate.Digital.vi"("Settings"="PWM Out 22.Settings") -> ("Output"=w486:bool)  [unwired: 10 in]
            n134 = call "PWM.Generate.Digital.vi"("Settings"="PWM Out 23.Settings") -> ("Output"=w485:bool)  [unwired: 10 in]
            n135 = call "PWM.Generate.Digital.vi"("Settings"="PWM Out 24.Settings") -> ("Output"=w484:bool)  [unwired: 10 in]
            n136 = call "PWM.Generate.Digital.vi"("Settings"="PWM Out 25.Settings") -> ("Output"=w483:bool)  [unwired: 10 in]
            n137 = call "PWM.Generate.Digital.vi"("Settings"="PWM Out 26.Settings") -> ("Output"=w482:bool)  [unwired: 10 in]
            n138 = call "PWM.Generate.Digital.vi"("Settings"="PWM Out 27.Settings") -> ("Output"=w481:bool)  [unwired: 10 in]
            n139 = Build Array(w247, w246, w245, w244, w243, w242, w241, w240) -> (w238:bool[])
            "Mod9.Monitor" <- w238
            n140 = call "PWM.Measure.Digital.vi"("State"=w470, "Settings"="PWM IN 3.Settings") -> ("Measurement"=→"PWM IN 3.Measure":T4)  [unwired: 8 in, 1 out]
            n141 = call "PWM.Measure.Digital.vi"("State"=w467, "Settings"="PWM IN 4.Settings") -> ("Measurement"=→"PWM IN 4.Measure":T4)  [unwired: 8 in, 1 out]
            n142 = call "PWM.Measure.Digital.vi"("State"=w464, "Settings"="PWM IN 5.Settings") -> ("Measurement"=→"PWM IN 5.Measure":T4)  [unwired: 8 in, 1 out]
            n143 = call "PWM.Measure.Digital.vi"("State"=w461, "Settings"="PWM IN 6.Settings") -> ("Measurement"=→"PWM IN 6.Measure":T4)  [unwired: 8 in, 1 out]
            n144 = Index Array(array=w352) -> (element #1=w350:bool, element #2=w347:bool, element #3=w344:bool, element #4=w341:bool, element #5=w338:bool, element #6=w335:bool, element #7=w332:bool, element #8=w329:bool, element #9=w326:bool, element #10=w323:bool, element #11=w320:bool, element #12=w317:bool, element #13=w314:bool, element #14=w311:bool, element #15=w308:bool, element #16=w305:bool, element #17=w302:bool, element #18=w299:bool, element #19=w296:bool, element #20=w293:bool, element #21=w290:bool, element #22=w287:bool, element #23=w284:bool, element #24=w281:bool, element #25=w278:bool, element #26=w275:bool, element #27=w272:bool, element #28=w269:bool, element #29=w266:bool, element #30=w263:bool, element #31=w260:bool, element #32=w257:bool)  [unwired: 32 in]
            n145 = Index Array(array=w434) -> (element #1=→"State 20":bool, element #2=→"State 21":bool, element #3=→"State 22":bool, element #4=→"State 23":bool, element #5=→"State 24":bool, element #6=→"State 25":bool, element #7=→"State 26":bool, element #8=→"State 27":bool, element #9=w424:bool, element #10=w421:bool, element #11=w418:bool, element #12=w415:bool, element #13=w412:bool, element #14=w409:bool, element #15=w406:bool, element #16=w403:bool, element #17=w400:bool, element #18=w397:bool, element #19=w394:bool, element #20=w391:bool, element #21=w388:bool, element #22=w385:bool, element #23=w382:bool, element #24=w379:bool, element #25=w376:bool, element #26=w373:bool, element #27=w370:bool, element #28=w367:bool, element #29=w364:bool, element #30=w361:bool, element #31=w358:bool, element #32=w355:bool)  [unwired: 32 in]
            n146 = call "Digital_Output_8Channels.vi"("States"=w238, "IO"=T27 {"DO 0"="Mod9/DO0", "DO 1"="Mod9/DO1", "DO 2"="Mod9/DO2", "DO 3"="Mod9/DO3", "DO 4"="Mod9/DO4", "DO 5"="Mod9/DO5", "DO 6"="Mod9/DO6", "DO 7"="Mod9/DO7"}) -> ()  [unwired: 1 in]
            n147 = Build Array(w507, w506, w505, w504, w503, w502, w501, w500, w499, w498, w497, w496, w495, w494, w493, w492, w491, w490, w489, w488, w487, w486, w485, w484, w483, w482, w481, "Output 0", "Output 1", "Output 2", "Output 3", "Output 4") -> (w474:bool[])
            "Mod3.Monitor" <- w474
            n148 = call "Static.Measure.Digital.vi"("State"=w350, "Settings"="State 52.Settings") -> ("Measurement"=→"State 52.Measure":T13)  [unwired: 9 in]
            n149 = call "Static.Measure.Digital.vi"("State"=w347, "Settings"="State 53.Settings") -> ("Measurement"=→"State 53.Measure":T13)  [unwired: 9 in]
            n150 = call "Static.Measure.Digital.vi"("State"=w344, "Settings"="State 54.Settings") -> ("Measurement"=→"State 54.Measure":T13)  [unwired: 9 in]
            n151 = call "Static.Measure.Digital.vi"("State"=w341, "Settings"="State 55.Settings") -> ("Measurement"=→"State 55.Measure":T13)  [unwired: 9 in]
            n152 = call "Static.Measure.Digital.vi"("State"=w338, "Settings"="State 56.Settings") -> ("Measurement"=→"State 56.Measure":T13)  [unwired: 9 in]
            n153 = call "Static.Measure.Digital.vi"("State"=w335, "Settings"="State 57.Settings") -> ("Measurement"=→"State 57.Measure":T13)  [unwired: 9 in]
            n154 = call "Static.Measure.Digital.vi"("State"=w332, "Settings"="State 58.Settings") -> ("Measurement"=→"State 58.Measure":T13)  [unwired: 9 in]
            n155 = call "Static.Measure.Digital.vi"("State"=w329, "Settings"="State 59.Settings") -> ("Measurement"=→"State 59.Measure":T13)  [unwired: 9 in]
            n156 = call "Static.Measure.Digital.vi"("State"=w326, "Settings"="State 60.Settings") -> ("Measurement"=→"State 60.Measure":T13)  [unwired: 9 in]
            n157 = call "Static.Measure.Digital.vi"("State"=w323, "Settings"="State 61.Settings") -> ("Measurement"=→"State 61.Measure":T13)  [unwired: 9 in]
            n158 = call "Static.Measure.Digital.vi"("State"=w320, "Settings"="State 62.Settings") -> ("Measurement"=→"State 62.Measure":T13)  [unwired: 9 in]
            n159 = call "Static.Measure.Digital.vi"("State"=w317, "Settings"="State 63.Settings") -> ("Measurement"=→"State 63.Measure":T13)  [unwired: 9 in]
            n160 = call "Static.Measure.Digital.vi"("State"=w314, "Settings"="State 64.Settings") -> ("Measurement"=→"State 64.Measure":T13)  [unwired: 9 in]
            n161 = call "Static.Measure.Digital.vi"("State"=w311, "Settings"="State 65.Settings") -> ("Measurement"=→"State 65.Measure":T13)  [unwired: 9 in]
            n162 = call "Static.Measure.Digital.vi"("State"=w308, "Settings"="State 66.Settings") -> ("Measurement"=→"State 66.Measure":T13)  [unwired: 9 in]
            n163 = call "Static.Measure.Digital.vi"("State"=w299, "Settings"="State 69.Settings") -> ("Measurement"=→"State 69.Measure":T13)  [unwired: 9 in]
            n164 = call "Static.Measure.Digital.vi"("State"=w296, "Settings"="State 70.Settings") -> ("Measurement"=→"State 70.Measure":T13)  [unwired: 9 in]
            n165 = call "Static.Measure.Digital.vi"("State"=w293, "Settings"="State 71.Settings") -> ("Measurement"=→"State 71.Measure":T13)  [unwired: 9 in]
            n166 = call "Static.Measure.Digital.vi"("State"=w290, "Settings"="State 72.Settings") -> ("Measurement"=→"State 72.Measure":T13)  [unwired: 9 in]
            n167 = call "Static.Measure.Digital.vi"("State"=w287, "Settings"="State 73.Settings") -> ("Measurement"=→"State 73.Measure":T13)  [unwired: 9 in]
            n168 = call "Static.Measure.Digital.vi"("State"=w284, "Settings"="State 74.Settings") -> ("Measurement"=→"State 74.Measure":T13)  [unwired: 9 in]
            n169 = call "Static.Measure.Digital.vi"("State"=w281, "Settings"="State 75.Settings") -> ("Measurement"=→"State 75.Measure":T13)  [unwired: 9 in]
            n170 = call "Static.Measure.Digital.vi"("State"=w278, "Settings"="State 76.Settings") -> ("Measurement"=→"State 76.Measure":T13)  [unwired: 9 in]
            n171 = call "Static.Measure.Digital.vi"("State"=w275, "Settings"="State 77.Settings") -> ("Measurement"=→"State 77.Measure":T13)  [unwired: 9 in]
            n172 = call "Static.Measure.Digital.vi"("State"=w272, "Settings"="State 78.Settings") -> ("Measurement"=→"State 78.Measure":T13)  [unwired: 9 in]
            n173 = call "Static.Measure.Digital.vi"("State"=w269, "Settings"="State 79.Settings") -> ("Measurement"=→"State 79.Measure":T13)  [unwired: 9 in]
            n174 = call "Static.Measure.Digital.vi"("State"=w266, "Settings"="State 80.Settings") -> ("Measurement"=→"State 80.Measure":T13)  [unwired: 9 in]
            n175 = call "Static.Measure.Digital.vi"("State"=w263, "Settings"="State 81.Settings") -> ("Measurement"=→"State 81.Measure":T13)  [unwired: 9 in]
            n176 = call "Static.Measure.Digital.vi"("State"=w260, "Settings"="State 82.Settings") -> ("Measurement"=→"State 82.Measure":T13)  [unwired: 9 in]
            n177 = call "Static.Measure.Digital.vi"("State"=w257, "Settings"="State 83.Settings") -> ("Measurement"=→"State 83.Measure":T13)  [unwired: 9 in]
            n178 = call "Static.Measure.Digital.vi"("State"=w305, "Settings"="State 67.Settings") -> ("Measurement"=→"State 67.Measure":T13)  [unwired: 9 in]
            n179 = call "Static.Measure.Digital.vi"("State"=w302, "Settings"="State 68.Settings") -> ("Measurement"=→"State 68.Measure":T13)  [unwired: 9 in]
            n180 = call "Static.Measure.Digital.vi"("State"=w424, "Settings"="State 28.Settings") -> ("Measurement"=→"State 28.Measure":T13)  [unwired: 9 in]
            n181 = call "Static.Measure.Digital.vi"("State"=w421, "Settings"="State 29.Settings") -> ("Measurement"=→"State 29.Measure":T13)  [unwired: 9 in]
            n182 = call "Static.Measure.Digital.vi"("State"=w418, "Settings"="State 30.Settings") -> ("Measurement"=→"State 30.Measure":T13)  [unwired: 9 in]
            n183 = call "Static.Measure.Digital.vi"("State"=w415, "Settings"="State 31.Settings") -> ("Measurement"=→"State 31.Measure":T13)  [unwired: 9 in]
            n184 = call "Static.Measure.Digital.vi"("State"=w412, "Settings"="State 32.Settings") -> ("Measurement"=→"State 32.Measure":T13)  [unwired: 9 in]
            n185 = call "Static.Measure.Digital.vi"("State"=w409, "Settings"="State 33.Settings") -> ("Measurement"=→"State 33.Measure":T13)  [unwired: 9 in]
            n186 = call "Static.Measure.Digital.vi"("State"=w406, "Settings"="State 34.Settings") -> ("Measurement"=→"State 34.Measure":T13)  [unwired: 9 in]
            n187 = call "Static.Measure.Digital.vi"("State"=w397, "Settings"="State 37.Settings") -> ("Measurement"=→"State 37.Measure":T13)  [unwired: 9 in]
            n188 = call "Static.Measure.Digital.vi"("State"=w394, "Settings"="State 38.Settings") -> ("Measurement"=→"State 38.Measure":T13)  [unwired: 9 in]
            n189 = call "Static.Measure.Digital.vi"("State"=w391, "Settings"="State 39.Settings") -> ("Measurement"=→"State 39.Measure":T13)  [unwired: 9 in]
            n190 = call "Static.Measure.Digital.vi"("State"=w388, "Settings"="State 40.Settings") -> ("Measurement"=→"State 40.Measure":T13)  [unwired: 9 in]
            n191 = call "Static.Measure.Digital.vi"("State"=w385, "Settings"="State 41.Settings") -> ("Measurement"=→"State 41.Measure":T13)  [unwired: 9 in]
            n192 = call "Static.Measure.Digital.vi"("State"=w382, "Settings"="State 42.Settings") -> ("Measurement"=→"State 42.Measure":T13)  [unwired: 9 in]
            n193 = call "Static.Measure.Digital.vi"("State"=w379, "Settings"="State 43.Settings") -> ("Measurement"=→"State 43.Measure":T13)  [unwired: 9 in]
            n194 = call "Static.Measure.Digital.vi"("State"=w376, "Settings"="State 44.Settings") -> ("Measurement"=→"State 44.Measure":T13)  [unwired: 9 in]
            n195 = call "Static.Measure.Digital.vi"("State"=w373, "Settings"="State 45.Settings") -> ("Measurement"=→"State 45.Measure":T13)  [unwired: 9 in]
            n196 = call "Static.Measure.Digital.vi"("State"=w370, "Settings"="State 46.Settings") -> ("Measurement"=→"State 46.Measure":T13)  [unwired: 9 in]
            n197 = call "Static.Measure.Digital.vi"("State"=w367, "Settings"="State 47.Settings") -> ("Measurement"=→"State 47.Measure":T13)  [unwired: 9 in]
            n198 = call "Static.Measure.Digital.vi"("State"=w364, "Settings"="State 48.Settings") -> ("Measurement"=→"State 48.Measure":T13)  [unwired: 9 in]
            n199 = call "Static.Measure.Digital.vi"("State"=w361, "Settings"="State 49.Settings") -> ("Measurement"=→"State 49.Measure":T13)  [unwired: 9 in]
            n200 = call "Static.Measure.Digital.vi"("State"=w358, "Settings"="State 50.Settings") -> ("Measurement"=→"State 50.Measure":T13)  [unwired: 9 in]
            n201 = call "Static.Measure.Digital.vi"("State"=w355, "Settings"="State 51.Settings") -> ("Measurement"=→"State 51.Measure":T13)  [unwired: 9 in]
            n202 = call "Static.Measure.Digital.vi"("State"=w403, "Settings"="State 35.Settings") -> ("Measurement"=→"State 35.Measure":T13)  [unwired: 9 in]
            n203 = call "Static.Measure.Digital.vi"("State"=w400, "Settings"="State 36.Settings") -> ("Measurement"=→"State 36.Measure":T13)  [unwired: 9 in]
            n204 = call "Digital_Output_32Channels.vi"("States"=w474, "IO"=T30 {"DO 0"="Mod3/DIO0", "DO 1"="Mod3/DIO1", "DO 2"="Mod3/DIO2", "DO 3"="Mod3/DIO3", "DO 4"="Mod3/DIO4", "DO 5"="Mod3/DIO5", "DO 6"="Mod3/DIO6", "DO 7"="Mod3/DIO7", "DO 8"="Mod3/DIO8", "DO 9"="Mod3/DIO9", "DO 10"="Mod3/DIO10", "DO 11"="Mod3/DIO11", "DO 12"="Mod3/DIO12", "DO 13"="Mod3/DIO13", "DO 14"="Mod3/DIO14", "DO 15"="Mod3/DIO15", "DO 16"="Mod3/DIO16", "DO 17"="Mod3/DIO17", "DO 18"="Mod3/DIO18", "DO 19"="Mod3/DIO19", "DO 20"="Mod3/DIO20", "DO 21"="Mod3/DIO21", "DO 22"="Mod3/DIO22", "DO 23"="Mod3/DIO23", "DO 24"="Mod3/DIO24", "DO 25"="Mod3/DIO25", "DO 26"="Mod3/DIO26", "DO 27"="Mod3/DIO27", "DO 28"="Mod3/DIO28", "DO 29"="Mod3/DIO29", "DO 30"="Mod3/DIO30", "DO 31"="Mod3/DIO31"}) -> ()  [unwired: 1 in]
            n205 = call "Loop.Timer.vi"("Loop Timer (uSec)"="Digital Loop Timer (uSec)") -> ("Actual Loop Period (usec)"=w641:u32)  [unwired: 10 in]
          }
          frame #1 {
            "Actual Digital Loop Period (usec)" <- w644
          }
        }
      }
      n206 = while "Analog Input Loop" {
        tunnel: w70 -> [w228]
        stop <- FALSE stop-if-true
        n207 = flat-sequence "Timing Control" {
          tunnel: w228 -> [w232]
          tunnel: [w232] -> w227
          tunnel: [w230] -> w226
          tunnel: w227 -> [_]
          tunnel: w226 -> [w233]
          frame #0 {
            n208 = call "Loop.Timer.vi"("Loop Timer (uSec)"="Analog Input Loop Timer (uSec)") -> ("Actual Loop Period (usec)"=w230:u32)  [unwired: 10 in]
          }
          frame #1 {
            "Actual Analog Input Loop Period (usec)" <- w233
          }
        }
      }
      n209 = while "Analog Output Loop" {
        tunnel: w70 -> [w220]
        stop <- FALSE stop-if-true
        n210 = flat-sequence "Timing Control" {
          tunnel: w220 -> [w224]
          tunnel: [w224] -> w219
          tunnel: [w222] -> w218
          tunnel: w219 -> [_]
          tunnel: w218 -> [w225]
          frame #0 {
            n211 = call "Loop.Timer.vi"("Loop Timer (uSec)"="Analog Output Loop Timer (uSec)") -> ("Actual Loop Period (usec)"=w222:u32)  [unwired: 10 in]
          }
          frame #1 {
            "Actual Analog Output Loop Period (usec)" <- w225
          }
        }
      }
      n212 = node-c288() -> (w74:T22)  [unwired: 1 in]
      n213 = timed-loop "EST APU Loop" {
        timing: w72 -> [_]
        timing-out: [_] -> w71
        tunnel: w70 -> [w75]
        stop <- _ stop-if-true
        n214 = call "Angle Processing Unit.vi"("settings.<user name>"="settings.apu 1", "register bus"=w75, "input.<user name>"="input.apu 1") -> ("output.<user name>"=→"output.apu 1":T17)  [unwired: 8 in]
      }
      n215 = timed-loop "Digital High Speed Loop" {
        timing: w74 -> [_]
        timing-out: [_] -> w73
        tunnel: w70 -> [w87]
        tunnel: w69 -> [w86]
        tunnel: w68 -> [w85]
        tunnel: w67 -> [w84]
        tunnel: w66 -> [w83]
        stop <- _ stop-if-true
        n216 = flat-sequence "Timing Control" {
          tunnel: w87 -> [w141]
          tunnel: w86 -> [w142]
          tunnel: w85 -> [w138]
          tunnel: w84 -> [w132]
          tunnel: w83 -> [w129]
          frame #0 {
            n217 = call "Directional Speed Sensor.vi"("load data"=w129, "settings.<user name>"="settings.Crank", "register bus"=w141, "input.<user name>"="input.Crank") -> ("digial output"=w122:bool)  [unwired: 7 in]
            n218 = call "Digital_Input_4Channels.vi"("IO"=T26 {"DI 0"="Mod2/DIO0", "DI 1"="Mod2/DIO1", "DI 2"="Mod2/DIO2", "DI 3"="Mod2/DIO3"}) -> ("States"=w118:bool[])
            "Mod2.Monitor" <- w118
            n219 = call "Digital Pattern Generation.vi"("load data"=w142, "settings.<user name>"="settings.Intake CAM 1", "register bus"=w141, "input.<user name>"="input.Intake CAM 1") -> ("digial output"=w126:bool)  [unwired: 7 in]
            n220 = call "Digital Pattern Generation.vi"("load data"=w138, "settings.<user name>"="settings.Exhaust CAM 1", "register bus"=w141, "input.<user name>"="input.Exhaust CAM 1") -> ("digial output"=w125:bool)  [unwired: 7 in]
            n221 = call "Digital Pattern Generation.vi"("load data"=w132, "settings.<user name>"="settings.Crank_Temp", "register bus"=w141, "input.<user name>"="input.Crank_Temp") -> ("digial output"=w123:bool)  [unwired: 7 in]
            n222 = call "WSS.Generate.Digital.vi"("Settings"="Front Driver WS.Settings") -> ("Bit1"=w135:bool, "Bit0"=w136:bool)  [unwired: 8 in, 1 out]
            n223 = Index Array(array=w118) -> (element #1=w116:bool, element #2=w113:bool, element #3=w110:bool, element #4=w98:bool)  [unwired: 4 in]
            n224 = call "PWM.Generate.Digital.vi"("Settings"="PWM Out 1.Settings") -> ("Output"=w128:bool)  [unwired: 10 in]
            n225 = call "PWM.Generate.Digital.vi"("Settings"="PWM Out 2.Settings") -> ("Output"=w127:bool)  [unwired: 10 in]
            n226 = call "PWM.Measure.Digital.vi"("State"=w116, "Settings"="PWM IN 1.Settings") -> ("Measurement"=→"PWM IN 1.Measure":T4)  [unwired: 8 in, 1 out]
            n227 = call "PWM.Measure.Digital.vi"("State"=w113, "Settings"="PWM IN 2.Settings") -> ("Measurement"=→"PWM IN 2.Measure":T4)  [unwired: 8 in, 1 out]
            n228 = call-poly "Measure Events.vi"("settings.<user name>"="settings.Cyl Inj 1", "register bus"=w141, "event"=w110) -> ("measured data"=w107:T35, "status.<user name>"=→"status.Cyl Inj 1":T2)  [unwired: 7 in]
            n229 = Build Array(w136, w135) -> (w124:bool[])
            n230 = call-poly "Measure Events.vi"("settings.<user name>"="settings.Cyl Inj 2", "register bus"=w141, "event"=w98) -> ("measured data"=w95:T35, "status.<user name>"=→"status.Cyl Inj 2":T2)  [unwired: 7 in]
            n231 = Build Array (concatenate)(w128, w127, w126, w125, w124, w123, w122) -> (w120:bool[])
            "Mod1.Monitor" <- w120
            n232 = call "Capture Event.vi"("event # to capture"=T25 1, "measured data"=w107) -> ("capture.<user name>"=→"capture.Cyl Inj 1.Event 1":T1)  [unwired: 9 in]
            n233 = call "Capture Event.vi"("event # to capture"=T25 2, "measured data"=w107) -> ("capture.<user name>"=→"capture.Cyl Inj 1.Event 2":T1)  [unwired: 9 in]
            n234 = call "Capture Event.vi"("event # to capture"=T25 3, "measured data"=w107) -> ("capture.<user name>"=→"capture.Cyl Inj 1.Event 3":T1)  [unwired: 9 in]
            n235 = call "Capture Event.vi"("event # to capture"=T25 4, "measured data"=w107) -> ("capture.<user name>"=→"capture.Cyl Inj 1.Event 4":T1)  [unwired: 9 in]
            n236 = call "Capture Event.vi"("event # to capture"=T25 1, "measured data"=w95) -> ("capture.<user name>"=→"capture.Cyl Inj 2.Event 1":T1)  [unwired: 9 in]
            n237 = call "Capture Event.vi"("event # to capture"=T25 2, "measured data"=w95) -> ("capture.<user name>"=→"capture.Cyl Inj 2.Event 2":T1)  [unwired: 9 in]
            n238 = call "Capture Event.vi"("event # to capture"=T25 3, "measured data"=w95) -> ("capture.<user name>"=→"capture.Cyl Inj 2.Event 3":T1)  [unwired: 9 in]
            n239 = call "Capture Event.vi"("event # to capture"=T25 4, "measured data"=w95) -> ("capture.<user name>"=→"capture.Cyl Inj 2.Event 4":T1)  [unwired: 9 in]
            n240 = call "Digital_Output_8Channels.vi"("States"=w120, "IO"=T27 {"DO 0"="Mod1/DIO0", "DO 1"="Mod1/DIO1", "DO 2"="Mod1/DIO2", "DO 3"="Mod1/DIO3", "DO 4"="Mod1/DIO4", "DO 5"="Mod1/DIO5", "DO 6"="Mod1/DIO6", "DO 7"="Mod1/DIO7"}) -> ()  [unwired: 1 in]
          }
        }
      }
      n241 = node-c288 ("Output Node")(w71) -> ()
      n242 = node-c288 ("Output Node")(w73) -> ()
    }
  }
